vi "DSF.Memory.Buffer.Config.Get Channel Offsets.vi"(8 "error in (no error)":errorcluster, 11 "Buffer Config in":refnum<class "DSF.Memory.Buffer.Config.lvclass">) -> (0 "error out":errorcluster, 2 "channel offsets ptr":refnum<class "DSF.Memory.Pointer.U64.lvclass">, 3 "Buffer Config out":refnum<class "DSF.Memory.Buffer.Config.lvclass">)   [LabVIEW 2016, in "DSF.Memory.lvlib" / "DSF.Memory.Buffer.Config.lvclass"]
uses:
  DSF.Memory.Buffer.Config.lvclass
  Memory.Pointer.U64/DSF.Memory.Pointer.U64.lvclass
  DSF.Memory.Buffer.Config.lvclass/DSF.Memory.Buffer.Config.ctl
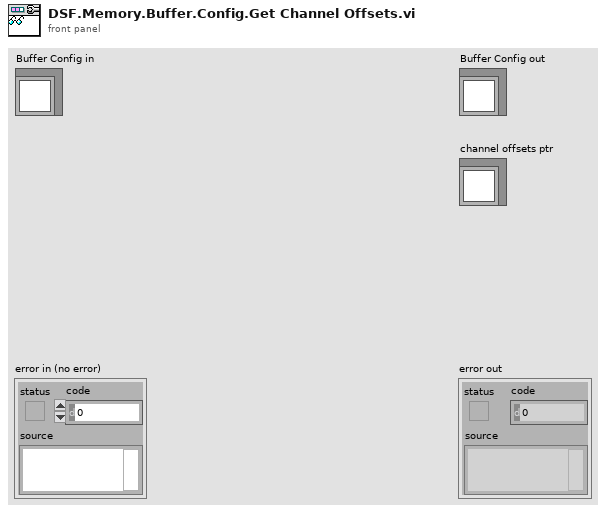
[diagram p1: front panel]
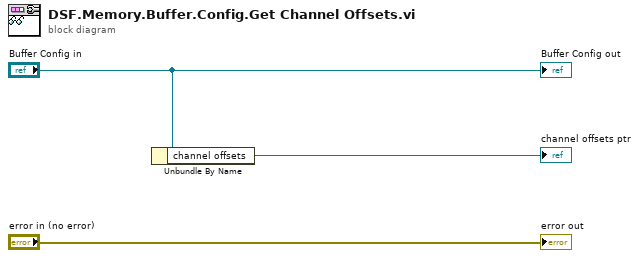
[diagram p0: block diagram]
diagram:
  n1 = Unbundle By Name("Buffer Config in") -> ("channel offsets"=→"channel offsets ptr":refnum<class "DSF.Memory.Pointer.U64.lvclass">)
  "error out" <- "error in (no error)"
  "Buffer Config out" <- "Buffer Config in"
